vi "Write Slew Rate.vi"(8 "error in":errorcluster, 10 "Slew Rate":dbl, 11 "3300 in":refnum<class "3300.lvclass">) -> (0 "error out":errorcluster, 3 "3300 out":refnum<class "3300.lvclass">)   [LabVIEW 2019, in "3300.lvlib" / "3300.lvclass"]
doc: "The 3300 does not throw an exception if an invalid slew rate is commanded. As a result we need to read back the slew rate and send it back the the UI so that the end user knows the eload coerced the slew rate."
uses:
  Library/3300.lvclass
  C:/Users/Public/Documents/Development/builds/Instruments/Electronic Load.lvlibp/Library/Electronic Load.lvclass
  builds/Instruments/Electronic Load.lvlibp/Accessors/Read Active Channel.vi
  builds/Instruments/Electronic Load.lvlibp/Accessors/Settings/Read Mode.vi
  builds/Instruments/Electronic Load.lvlibp/Library/Electronic Load.lvclass
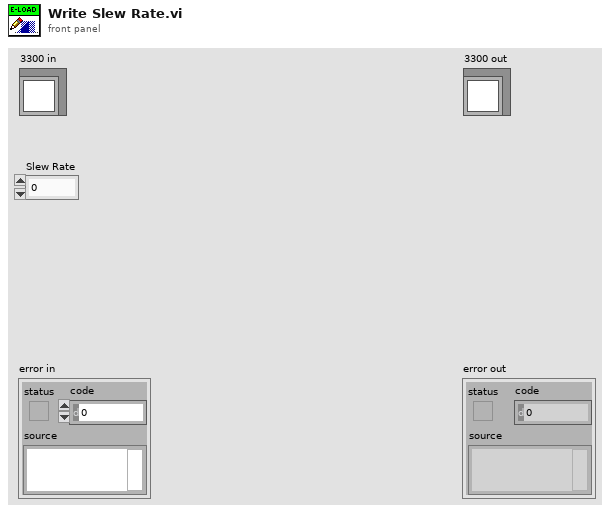
[diagram p1: front panel]
types:
  T1 = typedef "Electronic Load.lvlibp/Electronic Load.lvclass/E-Load Mode.ctl" = enum16{"Current", "Resistance", "Voltage"}
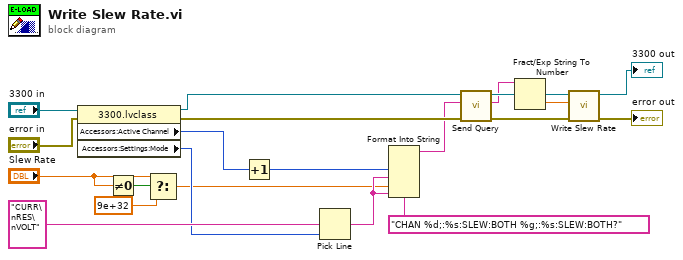
[diagram p0: block diagram]
diagram:
  n1 = property class="3300.lvclass"(reference="3300 in", error in="error in") -> (reference out=w14:refnum<class "3300.lvclass">, error out=w12:errorcluster, "Accessors:Active Channel"=w7:u32, "Accessors:Settings:Mode"=w8:T1)
  n2 = Not Equal To 0?(x="Slew Rate") -> (x != 0?=w4:bool)
  n3 = Select(t="Slew Rate", s=w4, f=9e+32) -> (s? t:f=w2:dbl)
  n4 = Increment(x=w7) -> (x+1=w6:u32)
  n5 = Pick Line(multi-line string="CURR\nRES\nVOLT" ("input 1"), line index=w8) -> (output string=w15:string)  [unwired: 1 in]
  n6 = Format Into String(format string="CHAN %d;:%s:SLEW:BOTH %g;:%s:SLEW:BOTH?", w6, w15, w2, w15) -> (resulting string=w9:string)  [unwired: 2 in, 1 out]
  n7 = call "Send Query.vi"("error in"=w12, "Query"=w9, "3300 in"=w14) -> ("error out"=w11:errorcluster, "Read Data"=w5:string, "3300 out"=w13:refnum<class "3300.lvclass">)  [unwired: 6 in]
  n8 = Fract/Exp String To Number(string=w5) -> (number=w10:dbl)  [unwired: 3 in, 1 out]
  n9 = call-parent "Write Slew Rate.vi"("error in"=w11, "Slew Rate"=w10, "Electronic Load in"=w13) -> ("error out"=→"error out":errorcluster, "Electronic Load out"=→"3300 out":refnum<class "3300.lvclass">)  [unwired: 7 in]
